vi "Msg Loop.vi"(11 "Self Actor in":refnum<class "Self Actor.lvclass">) -> ()   [LabVIEW 2021, in "AAM.lvlib" / "Self Actor.lvclass"]
uses:
  Self Actor.lvclass
  C:/PPLs/LabVIEW-Composed-Actor-Model-LVCAM/LabVIEW-Composed-Actor-Model-LVCAM/AAM/AAM/Actor/Actor.lvclass
  Self Actor.lvclass/Self Actor.ctl
  Msg/Msg.lvclass
  Msg Q/Msg Q.lvclass
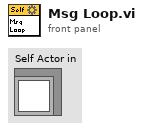
[diagram p1: front panel]
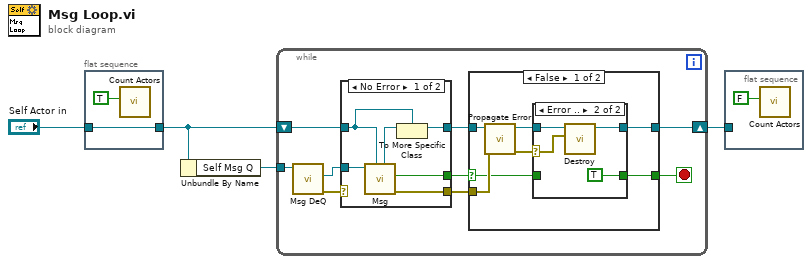
[diagram p0: block diagram]
diagram:
  n1 = flat-sequence {
    tunnel: "Self Actor in" -> [w6]
    tunnel: [w6] -> w2
    frame #0 {
      n2 = call "Count Actors.vi"("Increment?"=TRUE) -> ()  [unwired: 11 in]
    }
  }
  n3 = Unbundle By Name(w2) -> ("Self Msg Q"=w4:refnum<class "Msg Q.lvclass">)
  n4 = while {
    shift-right: [w10] -> w1
    shift-left: w2 -> [w15]
    tunnel: w4 -> [w7]
    stop <- w8 stop-if-true
    n5 = call "Msg DeQ.vi"("Msg Queue in"=w7) -> ("error out"=w13:errorcluster, "Msg"=w14:refnum<class "Msg.lvclass">)  [unwired: 9 in]
    n6 = case shown="No Error" w13 {
      selector: w13 -> [_ w37]
      tunnel: [w36 _] -> w12
      tunnel: [w35 w37] -> w11
      tunnel: [w32 w38] -> w9
      tunnel: w15 -> [w31 w38]
      tunnel: w14 -> [w34 _]
      frame No Error {
        n7 = call-dynamic "Msg.vi"("Actor in"=w31, "Msg in"=w34) -> ("error out"=w35:errorcluster, "Destroy Self?"=w36:bool, "Actor out"=w33:refnum<class "Actor.lvclass">)  [unwired: 7 in]
        n8 = To More Specific Class(target class=w31, reference=w33) -> (specific class reference=w32:refnum<class "Self Actor.lvclass">)  [unwired: 1 in, 1 out]
      }
      frame Error {
      }
    }
    n9 = case shown="False" w12 {
      selector: w12 -> [w16 w29]
      tunnel: w11 -> [w21 _]
      tunnel: [w19 w30] -> w10
      tunnel: w9 -> [w22 w30]
      tunnel: [w17 w29] -> w8
      frame False {
        n10 = call-dynamic "Propagate Error.vi"("error in (no error)"=w21, "Self Actor in"=w22) -> ("error out"=w20:errorcluster, "Self Actor out"=w18:refnum<class "Self Actor.lvclass">)  [unwired: 8 in]
        n11 = case shown="Error .." w20 {
          selector: w20 -> [_ w26]
          tunnel: [w24 w27] -> w19
          tunnel: w18 -> [w24 w28]
          tunnel: [w23 TRUE] -> w17
          tunnel: w16 -> [w23 _]
          frame No Error {
          }
          frame Error {
            n12 = call-dynamic "Destroy.vi"("Error"=w26, "Self Actor in"=w28) -> ("Self Actor out"=w27:refnum<class "Self Actor.lvclass">)  [unwired: 8 in, 1 out]
          }
        }
      }
      frame True {
      }
    }
  }
  n13 = flat-sequence {
    tunnel: w1 -> [_]
    frame #0 {
      n14 = call "Count Actors.vi"("Increment?"=FALSE) -> ()  [unwired: 11 in]
    }
  }
